vi "LD_PLCModbus Status.vi"(10 "Insert":i32, 11 "Enum":T1) -> ()   [LabVIEW 2019]
uses:
  Ctrl/123.ctl
panel:
  out "Input Registers":u16[](array[numeric])
  out "Read":u16
  in  "WriteStatus":u16
  in  "Numeric":u16
  out "Discrete Inputs":bool[](array[boolean])
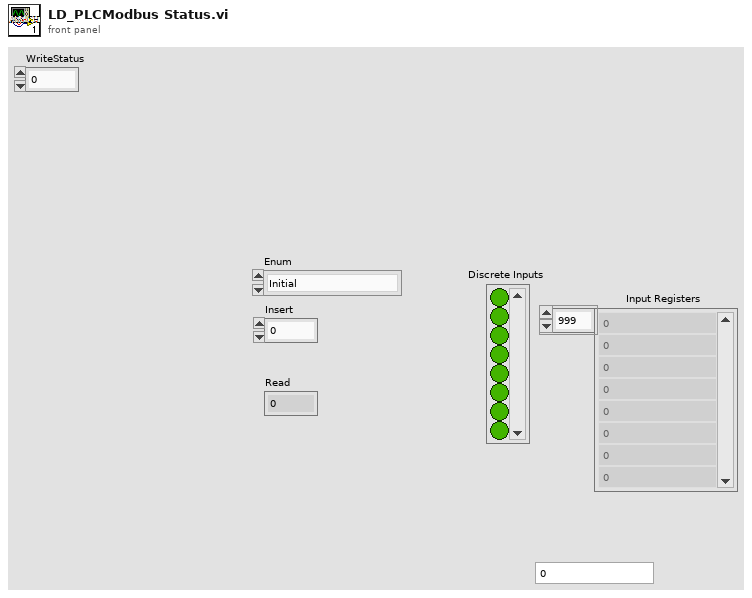
[diagram p1: front panel]
types:
  T1 = typedef "123.ctl" = enum16{"Initial", "Write", "Read"}
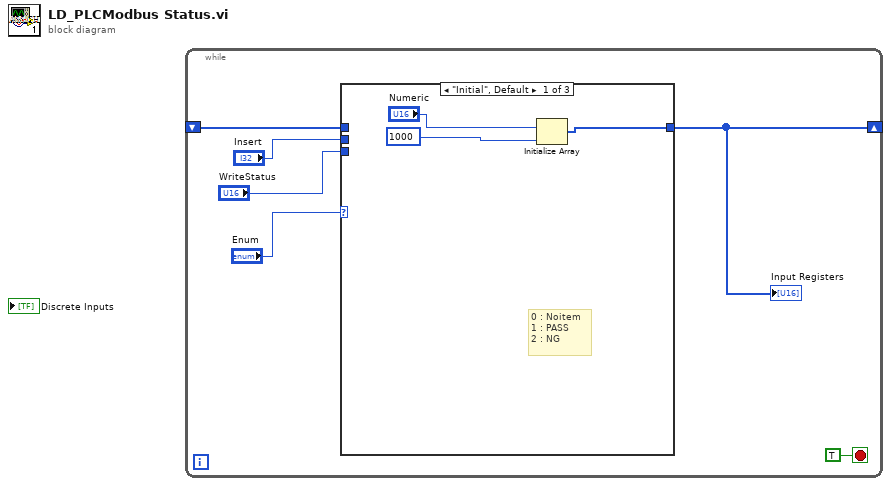
[diagram p0: block diagram]
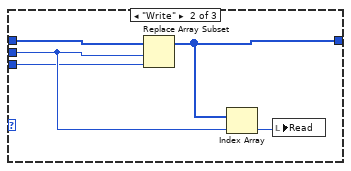
[diagram p2: hidden frame]
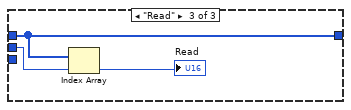
[diagram p3: hidden frame]
diagram:
  n1 = while {
    shift-right: [w1] -> _
    shift-left: _ -> [w5]
    stop <- TRUE stop-if-true
    n2 = case shown="\"Initial\", Default" "Enum" {
      tunnel: w5 -> [_ w14 w17]
      tunnel: [w8 w12 w17] -> w1
      tunnel: "Insert" -> [_ w13 w16]
      tunnel: "WriteStatus" -> [_ w11 _]
      frame "Initial", Default {
        # "0 : Noitem\n1 : PASS\n2 : NG"
        n3 = Initialize Array("Numeric", 1000 ("dimension size")) -> (w8:u16[])
      }
      frame "Write" {
        n4 = Replace Array Subset "Replace Array Subset"(array=w14, new element=w11, index=w13) -> (w12:u16[])
        n5 = Index Array(array=w12, index=w13) -> (element=w10:u16)
        n6 = local write "Read"(w10) -> ()
      }
      frame "Read" {
        n7 = Index Array(array=w17, index=w16) -> (element=→"Read":u16)
      }
    }
    "Input Registers" <- w1
  }
